vi "Read MainRef.vi"(8 "error in (no error)":errorcluster, 11 "RQMHModule in":refnum<class "Module.lvclass">) -> (0 "error out":errorcluster, 2 "MainRef":refnum<vi>, 3 "RQMHModule out":refnum<class "Module.lvclass">)   [LabVIEW 2024, in "Module.lvclass"]
uses:
  Module.lvclass
  Module.lvclass/Module.ctl
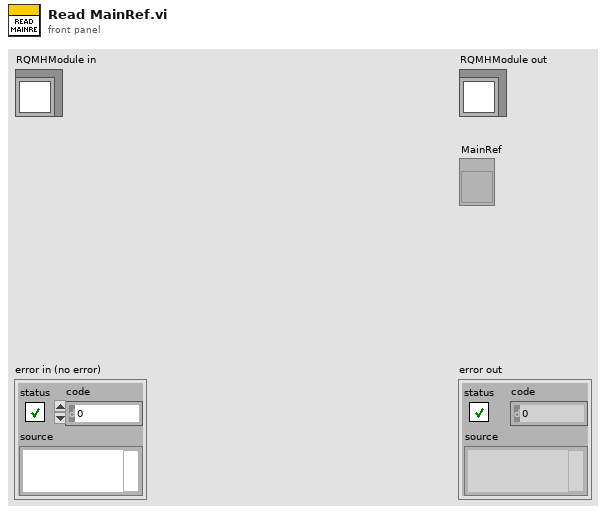
[diagram p1: front panel]
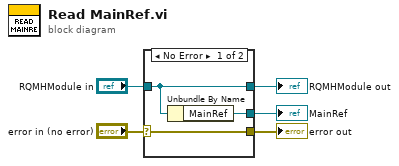
[diagram p0: block diagram]
diagram:
  n1 = case shown="No Error" "error in (no error)" {
    selector: "error in (no error)" -> [w8 w9]
    tunnel: [w8 w9] -> w4
    tunnel: [w7 w10] -> w2
    tunnel: "RQMHModule in" -> [w7 w10]
    tunnel: [w6 _] -> w1
    frame No Error {
      n2 = Unbundle By Name(w7) -> ("MainRef"=w6:refnum<vi>)
    }
    frame Error {
    }
  }
  "error out" <- w4
  "RQMHModule out" <- w2
  "MainRef" <- w1
